vi "Construct Actor Blocked Until Notified.vi"() -> (1 "Unblock Notifier":refnum<notifier>, 3 "ActorBlockedUntilNotified":refnum<class "ActorBlockedUntilNotified.lvclass">)   [LabVIEW 2017, in "ActorBlockedUntilNotified.lvclass"]
uses:
  ActorBlockedUntilNotified.lvclass
  ActorBlockedUntilNotified.lvclass/ActorBlockedUntilNotified.ctl
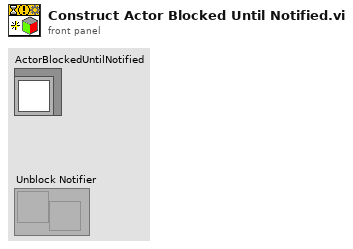
[diagram p1: front panel]
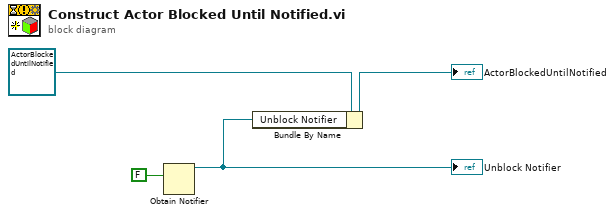
[diagram p0: block diagram]
diagram:
  n1 = Obtain Notifier(notification data type=FALSE) -> (notifier out=w1:refnum<notifier>)  [unwired: 3 in, 2 out]
  "Unblock Notifier" <- w1
  n2 = Bundle By Name(cluster=refnum<class "ActorBlockedUntilNotified.lvclass"> refnum ("ActorCountsMessageCycles.lvclass"), "Unblock Notifier"=w1) -> (→"ActorBlockedUntilNotified":refnum<class "ActorBlockedUntilNotified.lvclass">)
